vi "PowerSupply_ramp_or_hold.vi"(8 "error in (no error)":errorcluster, 11 "Mode":u16(ring) items=["Ramp to Setpoint", "Hold"]) -> (0 "error out":errorcluster)   [LabVIEW 2024]
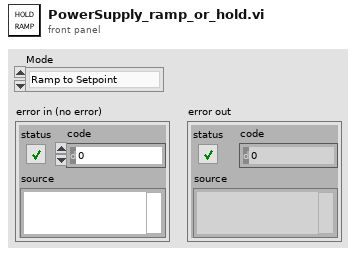
[diagram p1: front panel]
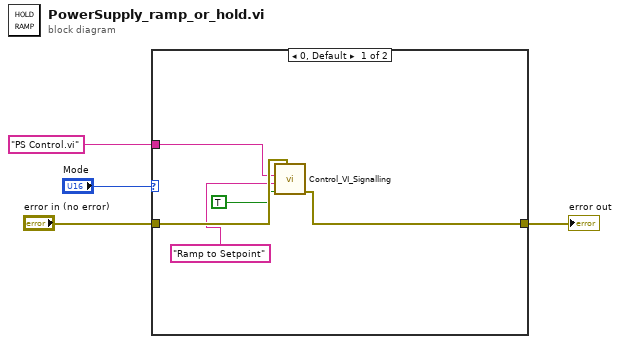
[diagram p0: block diagram]
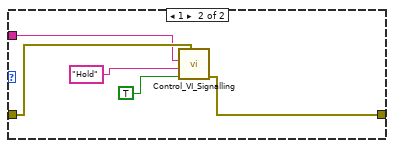
[diagram p2: hidden frame]
diagram:
  n1 = case shown="0, Default" "Mode" {
    tunnel: "error in (no error)" -> [w8 w14]
    tunnel: [w9 w10] -> w2
    tunnel: "PS Control.vi" ("Machine Name") -> [w5 w13]
    frame 0, Default {
      n2 = call "Control_VI_Signalling.vi"("error in (no error)"=w8, "Input Value"=TRUE, "Control Name"="Ramp to Setpoint", "Target VI name"=w5) -> ("error out"=w9:errorcluster)  [unwired: 7 in]
    }
    frame 1 {
      n3 = call "Control_VI_Signalling.vi"("error in (no error)"=w14, "Input Value"=TRUE, "Control Name"="Hold", "Target VI name"=w13) -> ("error out"=w10:errorcluster)  [unwired: 7 in]
    }
  }
  "error out" <- w2
